vi "Initialize.vi"(7 "timeout, ms (2000)":u32=2000, 8 "error in (no error)":errorcluster, 10 "baud rate (19200)":u32(ring)=19200 items=["300"=300, "600"=600, "1200"=1200, "2400"=2400, "4800"=4800, "9600"=9600, "19200"=19200, "38400"=38400, "76800"=76800, "115200"=115200], 11 "port":refnum<visa-resource-name>) -> (0 "error out":errorcluster, 3 "VI Probe out":refnum<class "PL MKS VI Probe.lvclass">)   [LabVIEW 2015, in "PL MKS VI Probe.lvclass"]
doc: "Initializes connection to device using specified settings."
uses:
  PL MKS VI Probe.lvclass
  PL MKS VI Probe.lvclass/PL MKS VI Probe.ctl
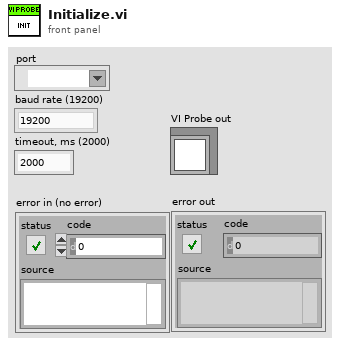
[diagram p1: front panel]
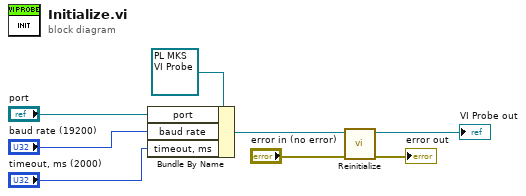
[diagram p0: block diagram]
diagram:
  n1 = Bundle By Name(cluster=refnum<class "PL MKS VI Probe.lvclass"> refnum, "port"="port", "baud rate"="baud rate (19200)", "timeout, ms"="timeout, ms (2000)") -> (w8:refnum<class "PL MKS VI Probe.lvclass">)
  n2 = call "Reinitialize.vi"("error in (no error)"="error in (no error)", "VI Probe in"=w8) -> ("error out"=→"error out":errorcluster, "VI Probe out"=→"VI Probe out":refnum<class "PL MKS VI Probe.lvclass">)  [unwired: 8 in]
